vi "Keithley 2636A - square current waveform.vi"() -> ()   [LabVIEW 2013]
uses:
  K2636/Keithley 2636A/Keithley/Public/Channel.ctl
  K2636/Keithley 2636A/Keithley/Keithley 2600 Series.lvlib
panel:
  out "Time per loop [ms]":u32=51
  out "Voltage ( V)":dbl=0.00457182 format="%#_6e"
  out "Current (A)":dbl=9.99963e-07 format="%#_6e"
  out "Time (s)":dbl=1.868
  in  "stop":bool
  in  "Node (0-64)":i8 min=0 max=64 step=1
  out "error out":errorcluster
  in  "Channel (Channel A)":T1
  in  "Error Query (False)":bool
  in  "error in (no error)":errorcluster
  in  "VISA resource name":refnum<visa-resource-name>="GPIB0::26::INSTR"
  out "Time per phase (ms)":dbl=500.0
  in  "Frequency (Hz)":dbl=1.0
  in  "Voltage  limit (V)":dbl=0.1
  in  "Current level (A)":dbl=1e-06
  out "Current (A)":cluster{dbl[], dbl[]}(graph)
  out "Voltage (V)":cluster{dbl[], dbl[]}(graph)
  # "Square waveform"
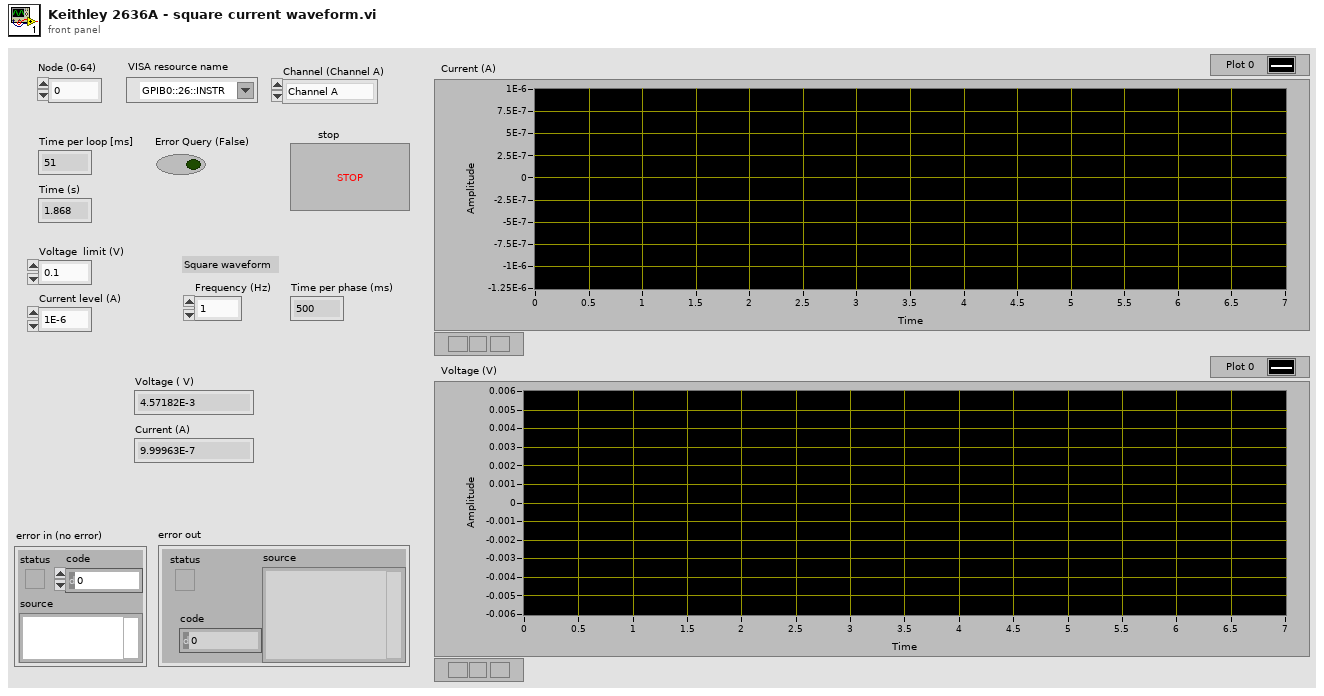
[diagram p1: front panel]
types:
  T1 = typedef "Keithley 2600 Series.lvlib/Channel.ctl" = enum32{"Channel A", "Channel B"}
  T2 = enum32{"Current", "Voltage", "IV", "Resistance", "Power"}
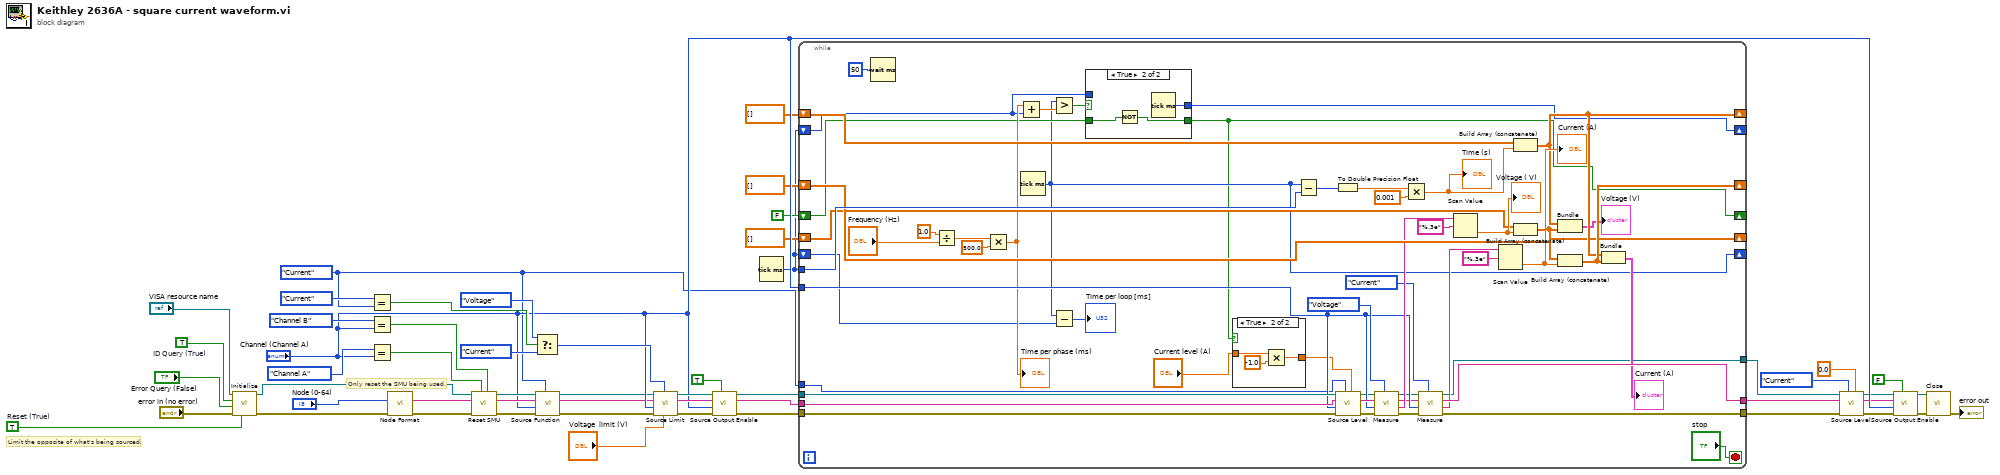
[diagram p0: block diagram]
diagram:
  w4 = enum32{"Current", "Voltage"}."Current" ("Source Function (Current)")
  w32 = TRUE  # Reset (True)
  w50 = TRUE  # ID Query (True)
  # "Limit the opposite of what's being sourced."
  # "Only reset the SMU being used."
  n1 = call "Initialize.vi"("Reset (True)"=w32, "error in (no error)"="error in (no error)", "Error Query (False)"="Error Query (False)", "ID Query (True)"=w50, "VISA resource name"="VISA resource name") -> ("error out"=w26:errorcluster, "VISA resource name out"=w48:refnum<visa-resource-name>)  [unwired: 1 in, 4 out]
  n2 = Equal?(x=enum32{"Current", "Voltage"}."Current", y=w4) -> (x = y?=w30:bool)
  n3 = Equal?(x=enum32{"Channel A", "Channel B"}."Channel B", y="Channel (Channel A)") -> (x = y?=w44:bool)
  n4 = Equal?(x=enum32{"Channel A", "Channel B"}."Channel A", y="Channel (Channel A)") -> (x = y?=w45:bool)
  n5 = call "Node Format.vi"("error in"=w26, "Node (0-64)"="Node (0-64)") -> ("error out"=w25:errorcluster, "Formatted Node"=w27:string)  [unwired: 8 out]
  n6 = call "Reset SMU.vi"("SMU B (No)"=w44, "SMU A (No)"=w45, "error in (no error)"=w25, "Node In"=w27, "VISA resource name"=w48) -> ("error out"=w43:errorcluster, "Node Out"=w41:string, "VISA resource name out"=w42:refnum<visa-resource-name>)  [unwired: 4 out]
  n7 = Select(t=enum32{"Current", "Voltage"}."Voltage" ("x"), s=w30, f=enum32{"Current", "Voltage"}."Current") -> (s? t:f=w28:enum32{"Current", "Voltage"})
  n8 = call "Source Function.vi"("Function (Current)"=w4, "error in (no error)"=w43, "Channel (Channel A)"="Channel (Channel A)", "Node In"=w41, "VISA resource name"=w42) -> ("error out"=w1:errorcluster, "Node Out"=w2:string, "VISA resource name out"=w3:refnum<visa-resource-name>)  [unwired: 4 out]
  n9 = call "Source Limit.vi"("Limit (0.000)"="Voltage  limit (V)", "Function (Current)"=w28, "error in (no error)"=w1, "Channel (Channel A)"="Channel (Channel A)", "Node In"=w2, "VISA resource name"=w3) -> ("error out"=w39:errorcluster, "Node Out"=w33:string, "VISA resource name out"=w40:refnum<visa-resource-name>)  [unwired: 3 out]
  n10 = call "Source Output Enable.vi"("Output (Off)"=TRUE, "error in (no error)"=w39, "Channel (Channel A)"="Channel (Channel A)", "Node In"=w33, "VISA resource name"=w40) -> ("error out"=w18:errorcluster, "Node Out"=w19:string, "VISA resource name out"=w20:refnum<visa-resource-name>)  [unwired: 4 out]
  n11 = Tick Count (ms)() -> (millisecond timer value=w5:u32)
  n12 = while {
    tunnel: "Channel (Channel A)" -> [w73]
    tunnel: w20 -> [w74]
    tunnel: w19 -> [w76]
    tunnel: w18 -> [w78]
    tunnel: w5 -> [w99]
    shift-right: [w81] -> _
    shift-left: dbl[] [] -> [w95]
    shift-right: [w80] -> _
    shift-left: dbl[] [] -> [w85]
    shift-right: [w83] -> _
    shift-left: dbl[] [] -> [w88]
    tunnel: [w60] -> w13
    tunnel: [w93] -> w7
    tunnel: [w92] -> w10
    shift-right: [w54] -> _
    shift-left: FALSE -> [w68]
    shift-right: [w71] -> _
    shift-left: w5 -> [w66]
    shift-right: [w56] -> _
    shift-left: w5 -> [w55]
    tunnel: w4 -> [w57]
    stop <- "stop" stop-if-true
    n13 = Wait (ms)(milliseconds to wait=u32 50) -> ()  [unwired: 1 out]
    n14 = Divide(x=1.0, y="Frequency (Hz)") -> (x/y=w101:dbl)
    n15 = Multiply(x=w101, y=500.0) -> (x*y=w70:dbl)
    "Time per phase (ms)" <- w70
    n16 = Add(x=w70, y=w66) -> (x+y=w67:dbl)
    n17 = Tick Count (ms)() -> (millisecond timer value=w56:u32)
    n18 = Greater?(x=w56, y=w67) -> (0:w69:bool)
    n19 = Subtract(x=w56, y=w55) -> (x-y=→"Time per loop [ms]":u32)
    n20 = case shown="True" w69 {
      tunnel: w66 -> [w107 _]
      tunnel: [w107 w110] -> w71
      tunnel: w68 -> [w106 w108]
      tunnel: [w106 w109] -> w54
      frame False {
      }
      frame True {
        n21 = Not(x=w108) -> (.not. x?=w109:bool)
        n22 = Tick Count (ms)() -> (millisecond timer value=w110:u32)
      }
    }
    n23 = case shown="True" w54 {
      tunnel: "Current level (A)" -> [w111 w113]
      tunnel: [w111 w114] -> w72
      frame False {
      }
      frame True {
        n24 = Multiply(x=w113, y=-1.0) -> (x*y=w114:dbl)
      }
    }
    n25 = Subtract(x=w56, y=w99) -> (x-y=w98:u32)
    n26 = To Double Precision Float(number=w98) -> (double precision float=w97:dbl)
    n27 = call "Source Level.vi"("Level (0.000)"=w72, "Function (Current)"=w57, "error in (no error)"=w78, "Channel (Channel A)"=w73, "Node In"=w76, "VISA resource name"=w74) -> ("error out"=w77:errorcluster, "Node Out"=w75:string, "VISA resource name out"=w59:refnum<visa-resource-name>)  [unwired: 3 out]
    n28 = call "Measure.vi"("Function (Current)"=T2."Voltage", "error in (no error)"=w77, "Channel (Channel A)"=w73, "Node In"=w75, "VISA resource name"=w59) -> ("error out"=w62:errorcluster, "Output"=w84:string, "Node Out"=w64:string, "VISA resource name out"=w63:refnum<visa-resource-name>)  [unwired: 2 in, 1 out]
    n29 = Multiply(x=w97, y=0.001) -> (x*y=w94:dbl)
    "Time (s)" <- w94
    n30 = call "Measure.vi"("Function (Current)"=T2."Current", "error in (no error)"=w62, "Channel (Channel A)"=w73, "Node In"=w64, "VISA resource name"=w63) -> ("error out"=w92:errorcluster, "Output"=w91:string, "Node Out"=w93:string, "VISA resource name out"=w60:refnum<visa-resource-name>)  [unwired: 2 in, 1 out]
    n31 = Scan Value(string=w84, format string="%.3e") -> (value=w86:dbl)  [unwired: 1 in, 1 out]
    "Voltage ( V)" <- w86
    n32 = Scan Value(string=w91, format string="%.3e") -> (value=w89:dbl)  [unwired: 1 in, 1 out]
    "Current (A)" <- w89
    n33 = Build Array (concatenate)(w95, w94) -> (w81:dbl[])
    n34 = Build Array (concatenate)(w85, w86) -> (w80:dbl[])
    n35 = Bundle(w81, w80) -> (→"Voltage (V)":cluster{dbl[], dbl[]})  [unwired: 1 in]
    n36 = Build Array (concatenate)(w88, w89) -> (w83:dbl[])
    n37 = Bundle(w81, w83) -> (→"Current (A)":cluster{dbl[], dbl[]})  [unwired: 1 in]
  }
  n38 = call "Source Level.vi"("Level (0.000)"=0.0, "Function (Current)"=enum32{"Current", "Voltage"}."Current", "error in (no error)"=w10, "Node In"=w7, "VISA resource name"=w13) -> ("error out"=w11:errorcluster, "Node Out"=w6:string, "VISA resource name out"=w12:refnum<visa-resource-name>)  [unwired: 1 in, 3 out]
  n39 = call "Source Output Enable.vi"("Output (Off)"=FALSE, "error in (no error)"=w11, "Channel (Channel A)"="Channel (Channel A)", "Node In"=w6, "VISA resource name"=w12) -> ("error out"=w38:errorcluster, "VISA resource name out"=w37:refnum<visa-resource-name>)  [unwired: 5 out]
  n40 = call "Close.vi"("error in (no error)"=w38, "VISA resource name"=w37) -> ("error out"=→"error out":errorcluster)  [unwired: 9 out]
